vi "Check If Network Error.vi"(11 "Error Code":i32) -> (3 "Network Error?":bool)   [LabVIEW 2012]
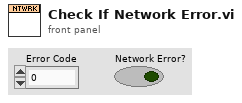
[diagram p1: front panel]
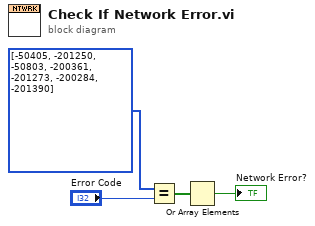
[diagram p0: block diagram]
diagram:
  n1 = Equal?(x=i32[] [-50405, -201250, -50803, -200361, -201273, -200284, -201390], y="Error Code") -> (x = y?=w1:bool[])
  n2 = Or Array Elements(Boolean array=w1) -> (logical OR=→"Network Error?":bool)
